vi "Read Window Name.vi"(8 "error in (no error)":errorcluster, 11 "Chat Window Controller in":refnum<class "Chat Window UI Controller.lvclass">) -> (0 "error out":errorcluster, 2 "Window Name":string, 3 "Chat Window Controller out":refnum<class "Chat Window UI Controller.lvclass">)   [LabVIEW 2020, in "Chat Window UI Controller.lvlib" / "Chat Window UI Controller.lvclass"]
uses:
  Chat Window UI Controller.lvclass
  Chat Window UI Controller.lvclass/Chat Window UI Controller.ctl
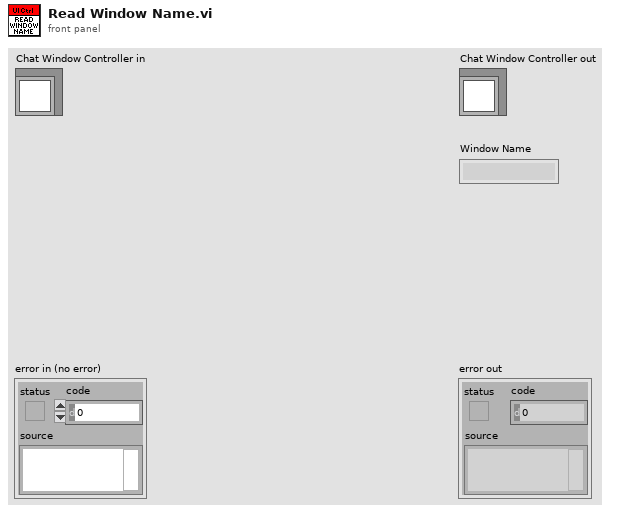
[diagram p1: front panel]
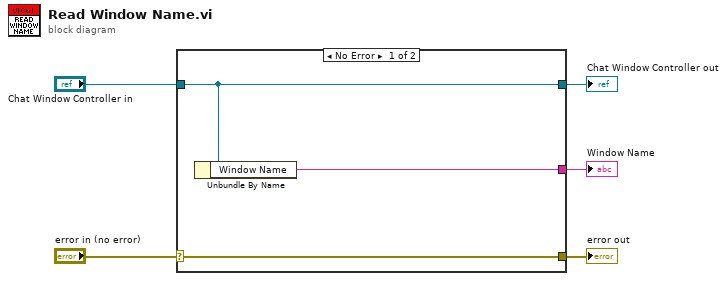
[diagram p0: block diagram]
diagram:
  n1 = case shown="No Error" "error in (no error)" {
    selector: "error in (no error)" -> [w8 w9]
    tunnel: [w8 w9] -> w4
    tunnel: [w7 w10] -> w2
    tunnel: "Chat Window Controller in" -> [w7 w10]
    tunnel: [w6 _] -> w1
    frame No Error {
      n2 = Unbundle By Name(w7) -> ("Window Name"=w6:string)
    }
    frame Error {
    }
  }
  "error out" <- w4
  "Chat Window Controller out" <- w2
  "Window Name" <- w1
